vi "GoV2.vi"(8 "Initial Coordinates":dbl[](array[numeric]), 9 "Timing Data":dbl[](array[numeric]), 10 "Control In":T1, 11 "CAD Dispense in":refnum<class "CAD Dispense.lvclass">) -> (2 "Control Out":T1, 3 "CAD Dispense Out":refnum<class "CAD Dispense.lvclass">)   [LabVIEW 2020, in "CAD Dispense.lvclass"]
uses:
  CAD Dispense.lvclass
  Aerotech.lvlib
  Program Files (x86)/Aerotech/A3200/LabVIEW/2010/Motion/MoveIncSingle.vi
  Controller/Dispenser/Dispenser.lvclass
  Program Files (x86)/Aerotech/A3200/LabVIEW/2010/Motion/WaitSingle.vi
  Controller/Motion/Motion.lvclass
  Controller/I-O/I-O.lvclass
  C:/Program Files (x86)/Aerotech/A3200/LabVIEW/2010/Bin/Aerotech.A3200.dll
  Program Files (x86)/Aerotech/A3200/LabVIEW/2010/Bin/Aerotech.A3200.dll
  Controller/Controllers.ctl
  Controller/Controller.lvclass
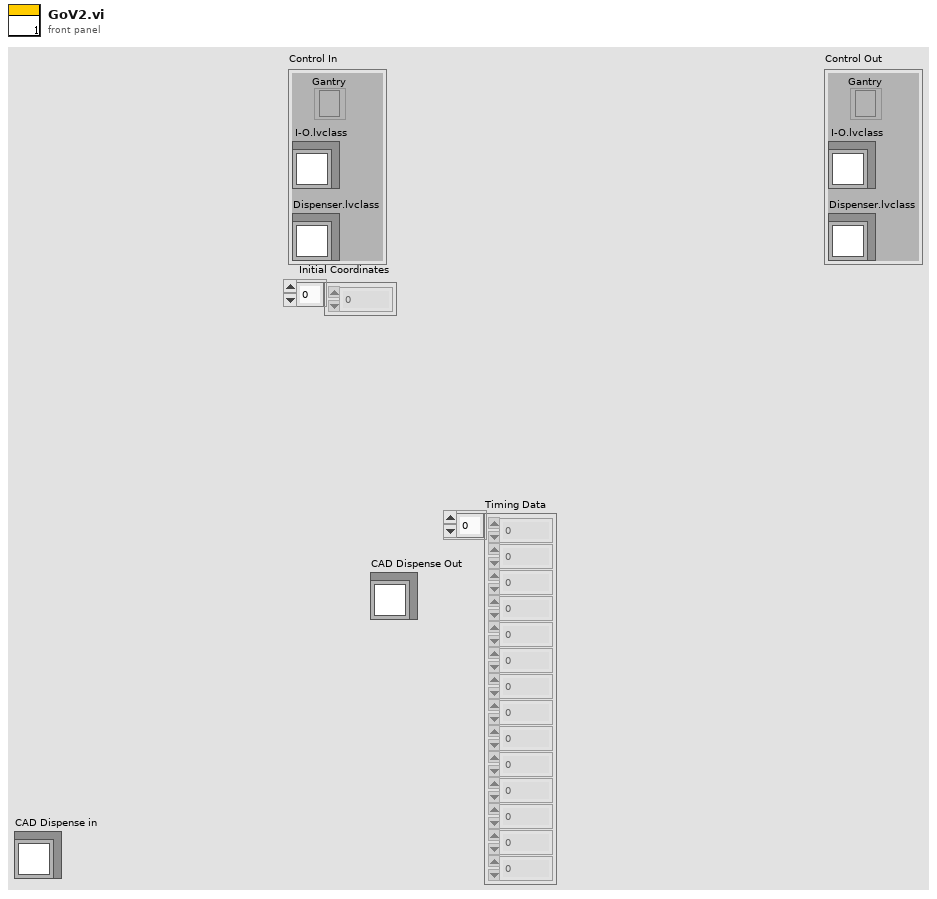
[diagram p1: front panel]
types:
  T1 = typedef "Controller.lvclass/Controllers.ctl" = cluster{"I-O.lvclass":refnum<class "I-O.lvclass">, "Dispenser.lvclass":refnum<class "Dispenser.lvclass">, "Gantry":refnum<k24>}
  T2 = cluster{"Motion":dbl[][], "Center":dbl[], "CW/CCW":dbl, "Dispense Type":enum16{"N-gon", "Square", "Arc", "Dot", "Line", "Circle"}}[]
  T3 = cluster{"Motion":dbl[][], "Center":dbl[], "CW/CCW":dbl, "Dispense Type":enum16{"N-gon", "Square", "Arc", "Dot", "Line", "Circle"}}
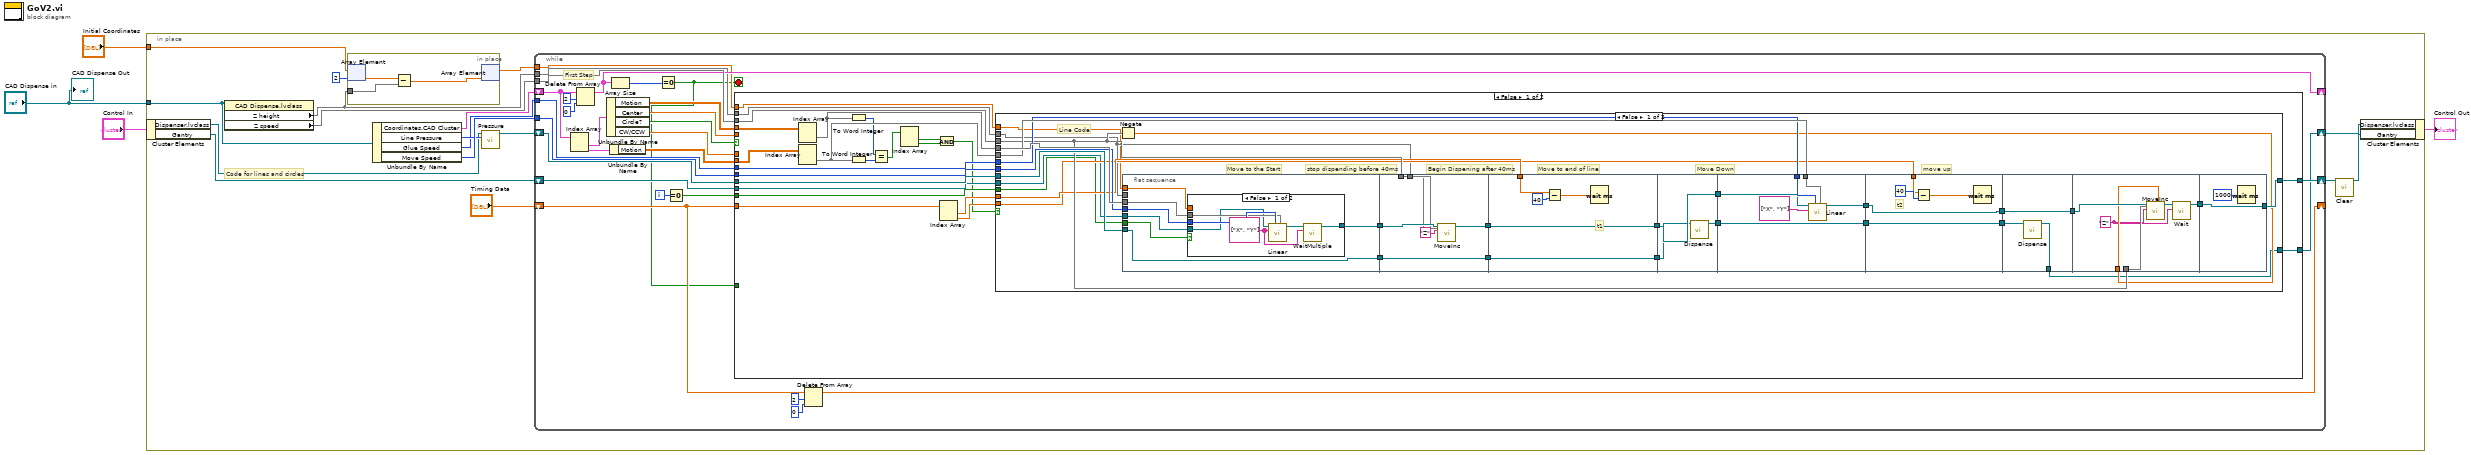
[diagram p0: block diagram]
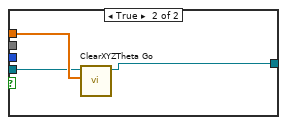
[diagram p2: hidden frame]
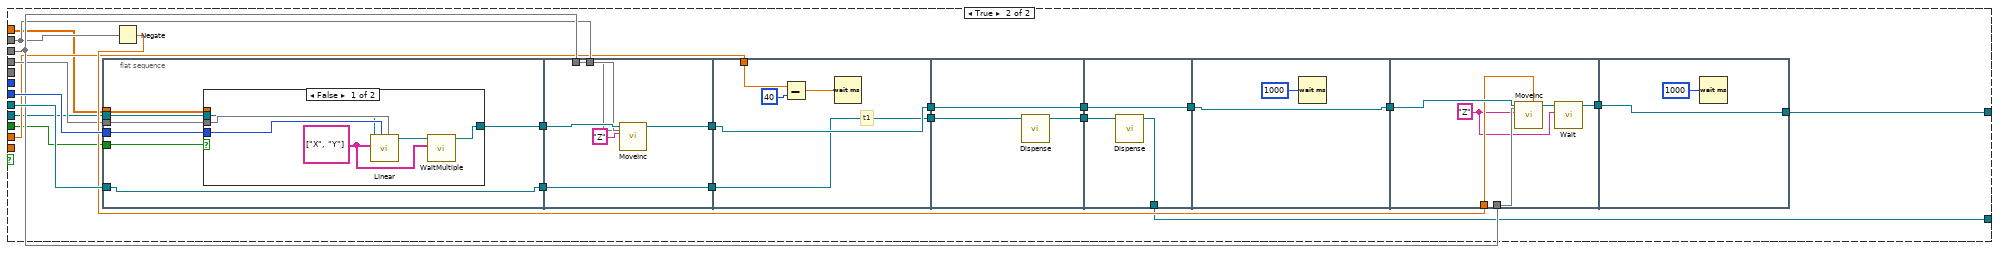
[diagram p3: hidden frame]
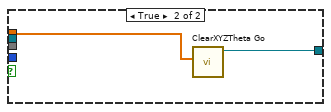
[diagram p4: hidden frame]
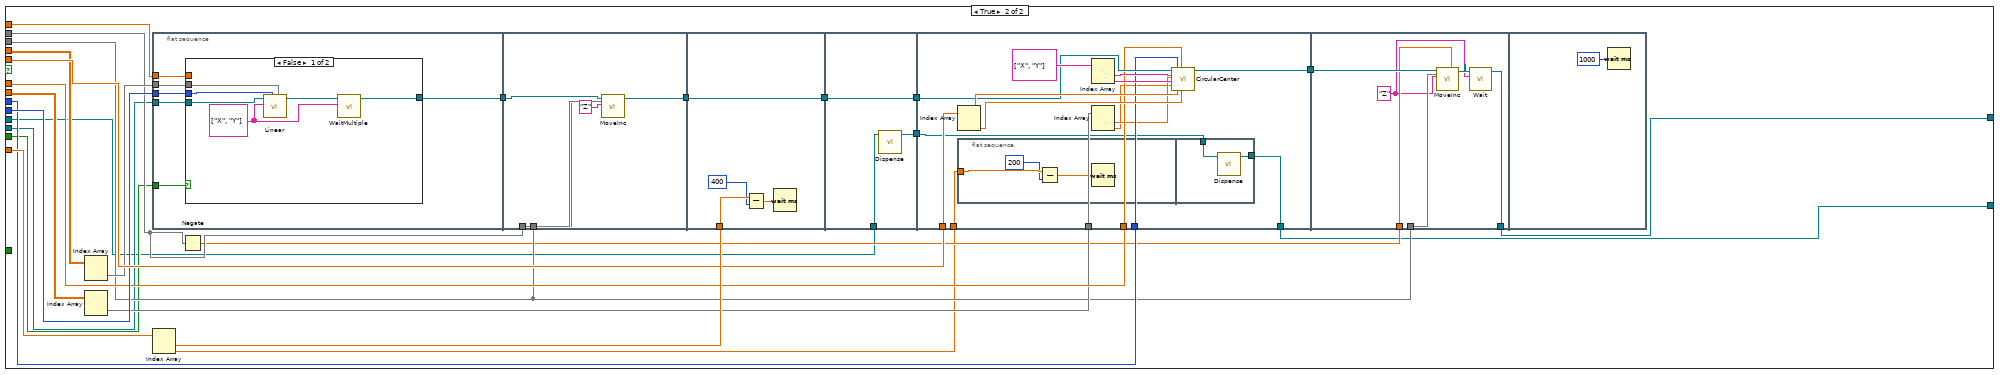
[diagram p5: hidden frame]
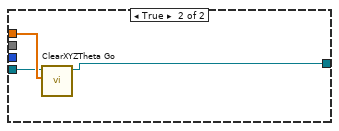
[diagram p6: hidden frame]
diagram:
  n1 = in-place {
    in-place-border: "CAD Dispense in" -> [w9]
    in-place-border: "Initial Coordinates" -> [w8]
    # "Code for lines and circles"
    n2 = in-place-cluster #1("Control In") -> ("Dispenser.lvclass"=w12:refnum<class "Dispenser.lvclass">, "Gantry"=w13:refnum<k24>)
    n3 = property class="CAD Dispense.lvclass"(reference=w9) -> ("Z height"=w7, "Z speed"=w16)  [unwired: 1 in, 2 out]
    n4 = in-place {
      in-place-border: w7 -> [w23]
      n5 = in-place-array #2(w8, 2) -> (w24:dbl)
      n6 = Subtract(x=w24, y=w23) -> (x-y=w22:dbl)
      n7 = in-place-array #2(w22) -> (w6:dbl[])  [unwired: 1 out]
    }
    n8 = Unbundle By Name "Unbundle By Name"(w9) -> ("Coordinates.CAD Cluster"=w19:T2, "Line Pressure"=w18:i64, "Glue Speed"=w15:i32, "Move Speed"=w21:i32)
    n9 = call-dynamic "Pressure.vi"("Pressure"=w18, "Dispenser in"=w12) -> ("Dispenser out"=w17:refnum<class "Dispenser.lvclass">)  [unwired: 8 in, 1 out]
    n10 = while {
      shift-right: [w31] -> w10
      shift-left: w17 -> [w47]
      tunnel: w21 -> [w50]
      shift-right: [w48] -> w14
      shift-left: w13 -> [w51]
      shift-right: [w41] -> _
      shift-left: "Timing Data" -> [w42]
      shift-right: [w37] -> _
      shift-left: w19 -> [w38]
      tunnel: w16 -> [w46]
      tunnel: w7 -> [w33]
      tunnel: w15 -> [w45]
      tunnel: w6 -> [w32]
      i -> [w35]
      stop <- w25 stop-if-true
      # "First Step"
      n11 = Index Array(array=w38) -> (element #1=w52:T3, element #2=w49:T3)  [unwired: 2 in]
      n12 = Delete From Array(array=w38, length=2, index=0) -> (array with subset deleted=w37:T2)  [unwired: 1 out]
      n13 = Unbundle By Name(w52) -> ("Motion"=w27:dbl[][], "Center"=w28:dbl[], "Circle?"=w30:bool, "CW/CCW"=w29:dbl)
      n14 = Unbundle By Name(w49) -> ("Motion"=w26:dbl[][])
      n15 = Array Size(array=w37) -> (size(s)=w36:i32)
      n16 = Equal To 0?(x=w36) -> (x = 0?=w25:bool)
      n17 = Equal To 0?(x=w35) -> (x = 0?=w34:bool)
      n18 = case shown="False" w30 {
        tunnel: w42 -> [w68 w239]
        tunnel: w28 -> [_ w246]
        tunnel: w27 -> [w61 w245]
        tunnel: w51 -> [w62 w226]
        tunnel: w50 -> [w72 w244]
        tunnel: w26 -> [w75 w235]
        tunnel: [w74 w222] -> w48
        tunnel: w47 -> [w73 w225]
        tunnel: w46 -> [w70 w233]
        tunnel: w33 -> [w71 w232]
        tunnel: w45 -> [w69 w237]
        tunnel: w29 -> [_ w236]
        tunnel: w34 -> [w65 w228]
        tunnel: w32 -> [w64 w230]
        tunnel: [w63 w223] -> w31
        tunnel: w25 -> [_ _]
        frame False {
          n19 = Index Array(array=w61) -> (element=w53:dbl[])  [unwired: 2 in]
          n20 = Index Array(array=w75) -> (element=w60:dbl[])  [unwired: 2 in]
          n21 = To Word Integer(number=w53) -> (16bit integer=w59:i16[])
          n22 = To Word Integer(number=w60) -> (16bit integer=w58:i16[])
          n23 = Equal?(x=w59, y=w58) -> (x = y?=w57:bool[])
          n24 = Index Array(array=w57) -> (element #1=w56:bool, element #2=w55:bool)  [unwired: 2 in]
          n25 = And(x=w56, y=w55) -> (x .and. y?=w54:bool)
          n26 = Index Array(array=w68) -> (element #1=w67:dbl, element #2=w66:dbl)  [unwired: 2 in]
          n27 = case shown="False" w54 {
            tunnel: w53 -> [w104 w162]
            tunnel: w60 -> [w103 _]
            tunnel: [w94 w172] -> w74
            tunnel: w73 -> [w93 w171]
            tunnel: w72 -> [w86 w166]
            tunnel: w71 -> [w79 w164]
            tunnel: w70 -> [w84 w165]
            tunnel: w69 -> [w85 _]
            tunnel: w67 -> [w82 w161]
            tunnel: w66 -> [w81 _]
            tunnel: w65 -> [w80 w160]
            tunnel: w64 -> [w78 w159]
            tunnel: [w77 w158] -> w63
            tunnel: w62 -> [w76 w157]
            frame False {
              # "Move to end of line"
              # "move up"
              # "stop dispending before 40ms"
              # "Begin Dispening after 40ms"
              # "Move Down"
              # "Move to the Start"
              # "Line Code"
              n28 = Negate(x=w84) -> (-x=w83:dbl)
              n29 = flat-sequence {
                tunnel: w104 -> [w110]
                tunnel: [w109] -> w102
                tunnel: w93 -> [w111]
                tunnel: [w111] -> w92
                tunnel: w86 -> [w108]
                tunnel: w80 -> [w106]
                tunnel: w79 -> [_]
                tunnel: w78 -> [w107]
                tunnel: w76 -> [w105]
                tunnel: w102 -> [w126]
                tunnel: [w125] -> w101
                tunnel: w92 -> [w124]
                tunnel: [w124] -> w91
                tunnel: w79 -> [w123]
                tunnel: w84 -> [w122]
                tunnel: w101 -> [w129]
                tunnel: [w129] -> w100
                tunnel: w91 -> [w128]
                tunnel: [w128] -> w90
                tunnel: w82 -> [w127]
                tunnel: w100 -> [w134]
                tunnel: [w134] -> w99
                tunnel: w90 -> [w133]
                tunnel: [w132] -> w89
                tunnel: w103 -> [w138]
                tunnel: w99 -> [w135]
                tunnel: [w139] -> w98
                tunnel: w89 -> [w140]
                tunnel: [w140] -> w88
                tunnel: w85 -> [w137]
                tunnel: w98 -> [w143]
                tunnel: [w143] -> w97
                tunnel: w88 -> [w142]
                tunnel: [w142] -> w87
                tunnel: w81 -> [w141]
                tunnel: w97 -> [w148]
                tunnel: [w148] -> w96
                tunnel: w87 -> [w147]
                tunnel: [w146] -> w77
                tunnel: w96 -> [w154]
                tunnel: [w152] -> w95
                tunnel: w84 -> [w151]
                tunnel: w83 -> [w150]
                tunnel: w95 -> [w155]
                tunnel: [w155] -> w94
                frame #0 {
                  n30 = case shown="False" w106 {
                    tunnel: [w116 w120] -> w109
                    tunnel: w110 -> [w113 _]
                    tunnel: w108 -> [w114 _]
                    tunnel: w107 -> [_ w119]
                    tunnel: w105 -> [w112 w118]
                    frame False {
                      w115 = string[] ["X", "Y"] ("axis names")
                      n31 = call "Linear.vi"("distances"=w113, "speed"=w114, "axis names"=w115, "controller in"=w112) -> ("controller out"=w117:refnum<k24>)  [unwired: 6 in, 1 out]
                      n32 = call "WaitMultiple.vi"("axis names"=w115, "controller in"=w117) -> ("controller out"=w116:refnum<k24>)  [unwired: 7 in, 2 out]
                    }
                    frame True {
                      n33 = call "ClearXYZTheta Go.vi"("XYZTheta In"=w119, "Gantry 2"=w118) -> ("Gantry 3"=w120:refnum<k24>)  [unwired: 7 in, 2 out]
                    }
                  }
                }
                frame #1 {
                  n34 = call-poly "MoveInc.vi"("distance"=w123, "speed"=w122, "axis name"="Z", "controller in"=w126) -> ("controller out"=w125:refnum<k24>)  [unwired: 6 in, 1 out]
                }
                frame #2 {
                  # "t1"
                  n35 = Subtract(x=w127, y=u32 40 ("milliseconds to wait")) -> (x-y=w130:dbl)
                  n36 = Wait (ms)(milliseconds to wait=w130) -> ()  [unwired: 1 out]
                }
                frame #3 {
                  n37 = call-dynamic "Dispense.vi"("Dispenser in"=w133) -> ("Dispenser out"=w132:refnum<class "Dispenser.lvclass">)  [unwired: 9 in, 1 out]
                }
                frame #4 {
                  n38 = call "Linear.vi"("distances"=w138, "speed"=w137, "axis names"=string[] ["X", "Y"], "controller in"=w135) -> ("controller out"=w139:refnum<k24>)  [unwired: 6 in, 1 out]
                }
                frame #5 {
                  # "t2"
                  n39 = Subtract(x=w141, y=40) -> (x-y=w144:dbl)
                  n40 = Wait (ms)(milliseconds to wait=w144) -> ()  [unwired: 1 out]
                }
                frame #6 {
                  n41 = call-dynamic "Dispense.vi"("Dispenser in"=w147) -> ("Dispenser out"=w146:refnum<class "Dispenser.lvclass">)  [unwired: 9 in, 1 out]
                }
                frame #7 {
                  w149 = "Z" ("axis name")
                  n42 = call-poly "MoveInc.vi"("distance"=w150, "speed"=w151, "axis name"=w149, "controller in"=w154) -> ("controller out"=w153:refnum<k24>)  [unwired: 6 in, 1 out]
                  n43 = call-poly "Wait.vi"("axis name"=w149, "controller in"=w153) -> ("controller out"=w152:refnum<k24>)  [unwired: 7 in, 2 out]
                }
                frame #8 {
                  n44 = Wait (ms)(milliseconds to wait=u32 1000) -> ()  [unwired: 1 out]
                }
              }
            }
            frame True {
              n45 = flat-sequence {
                tunnel: [w181] -> w179
                tunnel: w171 -> [w186]
                tunnel: [w186] -> w168
                tunnel: w166 -> [w183]
                tunnel: w162 -> [w184]
                tunnel: w160 -> [w185]
                tunnel: w159 -> [w182]
                tunnel: w157 -> [w180]
                tunnel: w179 -> [w200]
                tunnel: [w199] -> w178
                tunnel: [w198] -> w169
                tunnel: w168 -> [w198]
                tunnel: w164 -> [w197]
                tunnel: w165 -> [w196]
                tunnel: w178 -> [w203]
                tunnel: [w203] -> w177
                tunnel: [w202] -> w170
                tunnel: w169 -> [w202]
                tunnel: w161 -> [w201]
                tunnel: w177 -> [w208]
                tunnel: [w208] -> w174
                tunnel: w170 -> [w207]
                tunnel: [w206] -> w167
                tunnel: [w211] -> w175
                tunnel: w174 -> [w211]
                tunnel: w167 -> [w210]
                tunnel: [w209] -> w158
                tunnel: [w212] -> w176
                tunnel: w175 -> [w212]
                tunnel: w176 -> [w218]
                tunnel: [w217] -> w173
                tunnel: w165 -> [w216]
                tunnel: w163 -> [w215]
                tunnel: w173 -> [w220]
                tunnel: [w220] -> w172
                frame #0 {
                  n46 = case shown="False" w185 {
                    tunnel: [w191 w194] -> w181
                    tunnel: w183 -> [w188 _]
                    tunnel: w184 -> [w189 _]
                    tunnel: w182 -> [_ w193]
                    tunnel: w180 -> [w187 _]
                    frame False {
                      w190 = string[] ["X", "Y"] ("axis names")
                      n47 = call "Linear.vi"("distances"=w189, "speed"=w188, "axis names"=w190, "controller in"=w187) -> ("controller out"=w192:refnum<k24>)  [unwired: 6 in, 1 out]
                      n48 = call "WaitMultiple.vi"("axis names"=w190, "controller in"=w192) -> ("controller out"=w191:refnum<k24>)  [unwired: 7 in, 2 out]
                    }
                    frame True {
                      n49 = call "ClearXYZTheta Go.vi"("XYZTheta In"=w193) -> ("Gantry 3"=w194:refnum<k24>)  [unwired: 8 in, 2 out]
                    }
                  }
                }
                frame #1 {
                  n50 = call-poly "MoveInc.vi"("distance"=w197, "speed"=w196, "axis name"="Z", "controller in"=w200) -> ("controller out"=w199:refnum<k24>)  [unwired: 6 in, 1 out]
                }
                frame #2 {
                  # "t1"
                  n51 = Subtract(x=w201, y=u32 40 ("milliseconds to wait")) -> (x-y=w204:dbl)
                  n52 = Wait (ms)(milliseconds to wait=w204) -> ()  [unwired: 1 out]
                }
                frame #3 {
                  n53 = call-dynamic "Dispense.vi"("Dispenser in"=w207) -> ("Dispenser out"=w206:refnum<class "Dispenser.lvclass">)  [unwired: 9 in, 1 out]
                }
                frame #4 {
                  n54 = call-dynamic "Dispense.vi"("Dispenser in"=w210) -> ("Dispenser out"=w209:refnum<class "Dispenser.lvclass">)  [unwired: 9 in, 1 out]
                }
                frame #5 {
                  n55 = Wait (ms)(milliseconds to wait=u32 1000) -> ()  [unwired: 1 out]
                }
                frame #6 {
                  w214 = "Z" ("axis name")
                  n56 = call-poly "MoveInc.vi"("distance"=w215, "speed"=w216, "axis name"=w214, "controller in"=w218) -> ("controller out"=w219:refnum<k24>)  [unwired: 6 in, 1 out]
                  n57 = call-poly "Wait.vi"("axis name"=w214, "controller in"=w219) -> ("controller out"=w217:refnum<k24>)  [unwired: 7 in, 2 out]
                }
                frame #7 {
                  n58 = Wait (ms)(milliseconds to wait=u32 1000) -> ()  [unwired: 1 out]
                }
              }
              n59 = Negate(x=w164) -> (-x=w163:dbl)
            }
          }
        }
        frame True {
          n60 = Index Array(array=w245) -> (element=w238:dbl[])  [unwired: 2 in]
          n61 = Index Array(array=w235) -> (element=w234:dbl[])  [unwired: 2 in]
          n62 = flat-sequence {
            tunnel: w244 -> [w252]
            tunnel: w238 -> [w251]
            tunnel: w230 -> [w253]
            tunnel: [w250] -> w229
            tunnel: w228 -> [w249]
            tunnel: w226 -> [w248]
            tunnel: [w267] -> w243
            tunnel: w233 -> [w263]
            tunnel: w232 -> [w264]
            tunnel: w229 -> [w265]
            tunnel: w247 -> [w271]
            tunnel: w243 -> [w270]
            tunnel: [w270] -> w241
            tunnel: [w274] -> w242
            tunnel: w241 -> [w274]
            tunnel: w225 -> [w273]
            tunnel: [w272] -> w224
            tunnel: [w290] -> w240
            tunnel: w227 -> [w277]
            tunnel: w234 -> [w280]
            tunnel: w236 -> [w281]
            tunnel: w237 -> [w282]
            tunnel: w242 -> [w283]
            tunnel: w246 -> [w286]
            tunnel: w224 -> [w276]
            tunnel: [w275] -> w223
            tunnel: w240 -> [w301]
            tunnel: w233 -> [w299]
            tunnel: w231 -> [w298]
            tunnel: [w296] -> w222
            frame #0 {
              n63 = case shown="False" w249 {
                tunnel: [w258 w262] -> w250
                tunnel: w253 -> [_ w261]
                tunnel: w252 -> [w256 _]
                tunnel: w251 -> [w255 _]
                tunnel: w248 -> [w254 w260]
                frame False {
                  w257 = string[] ["X", "Y"] ("axis names")
                  n64 = call "Linear.vi"("distances"=w255, "speed"=w256, "axis names"=w257, "controller in"=w254) -> ("controller out"=w259:refnum<k24>)  [unwired: 6 in, 1 out]
                  n65 = call "WaitMultiple.vi"("axis names"=w257, "controller in"=w259) -> ("controller out"=w258:refnum<k24>)  [unwired: 7 in, 2 out]
                }
                frame True {
                  n66 = call "ClearXYZTheta Go.vi"("XYZTheta In"=w261, "Gantry 2"=w260) -> ("Gantry 3"=w262:refnum<k24>)  [unwired: 7 in, 2 out]
                }
              }
            }
            frame #1 {
              n67 = call-poly "MoveInc.vi"("distance"=w264, "speed"=w263, "axis name"="Z", "controller in"=w265) -> ("controller out"=w267:refnum<k24>)  [unwired: 6 in, 1 out]
            }
            frame #2 {
              n68 = Subtract(x=w271, y=u32 400 ("milliseconds to wait")) -> (x-y=w268:dbl)
              n69 = Wait (ms)(milliseconds to wait=w268) -> ()  [unwired: 1 out]
            }
            frame #3 {
              n70 = call-dynamic "Dispense.vi"("Dispenser in"=w273) -> ("Dispenser out"=w272:refnum<class "Dispenser.lvclass">)  [unwired: 9 in, 1 out]
            }
            frame #4 {
              n71 = Index Array "Index Array"(array=w286) -> (element #1=w285:dbl, element #2=w284:dbl)  [unwired: 2 in]
              n72 = flat-sequence {
                tunnel: w277 -> [w293]
                tunnel: w276 -> [w295]
                tunnel: [w294] -> w275
                frame #0 {
                  n73 = Subtract(x=w293, y=u32 200 ("milliseconds to wait")) -> (x-y=w292:dbl)
                  n74 = Wait (ms)(milliseconds to wait=w292) -> ()  [unwired: 1 out]
                }
                frame #1 {
                  n75 = call-dynamic "Dispense.vi"("Dispenser in"=w295) -> ("Dispenser out"=w294:refnum<class "Dispenser.lvclass">)  [unwired: 9 in, 1 out]
                }
              }
              n76 = Index Array(array=string[] ["X", "Y"]) -> (element #1=w289:string, element #2=w288:string)  [unwired: 2 in]
              n77 = Index Array(array=w280) -> (element #1=w279:dbl, element #2=w278:dbl)  [unwired: 2 in]
              n78 = call "CircularCenter.vi"("controller in"=w283, "axis 1 name"=w289, "axis 1 endpoint"=w279, "axis 2 name"=w288, "axis 2 endpoint"=w278, "speed"=w282, "axis 1 center point"=w285, "direction"=w281, "axis 2 center point"=w284) -> ("controller out"=w290:refnum<k24>)  [unwired: 9 in, 1 out]
            }
            frame #5 {
              w297 = "Z" ("axis name")
              n79 = call-poly "MoveInc.vi"("distance"=w298, "speed"=w299, "axis name"=w297, "controller in"=w301) -> ("controller out"=w300:refnum<k24>)  [unwired: 6 in, 1 out]
              n80 = call-poly "Wait.vi"("axis name"=w297, "controller in"=w300) -> ("controller out"=w296:refnum<k24>)  [unwired: 7 in, 2 out]
            }
            frame #6 {
              n81 = Wait (ms)(milliseconds to wait=u32 1000) -> ()  [unwired: 1 out]
            }
          }
          n82 = Index Array(array=w239) -> (element #1=w247:dbl, element #2=w227:dbl)  [unwired: 2 in]
          n83 = Negate(x=w232) -> (-x=w231:dbl)
        }
      }
      n84 = Delete From Array(array=w42, length=2, index=0) -> (array with subset deleted=w41:dbl[])  [unwired: 1 out]
    }
    n85 = call "Clear.vi"("Gantry 2"=w14) -> ("Gantry 3"=w11:refnum<k24>)  [unwired: 9 in, 1 out]
    n86 = in-place-cluster #1("Dispenser.lvclass"=w10, "Gantry"=w11) -> (→"Control Out":T1)
  }
  "CAD Dispense Out" <- "CAD Dispense in"
